vi "MDAQ_CalibrationCalcBlock.vi"(9 "threshold":dbl format="%0.2f", 10 "Spectrum":dbl[](array[numeric])) -> (1 "Mirror Fit":T1, 2 "Fit":T1, 4 "Spectrum Plot":cluster{cluster{dbl, dbl}[]}[](array[cluster]), 6 "Fitted Plots":cluster{dbl[], dbl[]}[](array[cluster]))   [LabVIEW 2021]
uses:
  <vilib>/Analysis/NI_AALPro.lvlib
  <vilib>/Analysis/NI_AAL_SigProc.lvlib
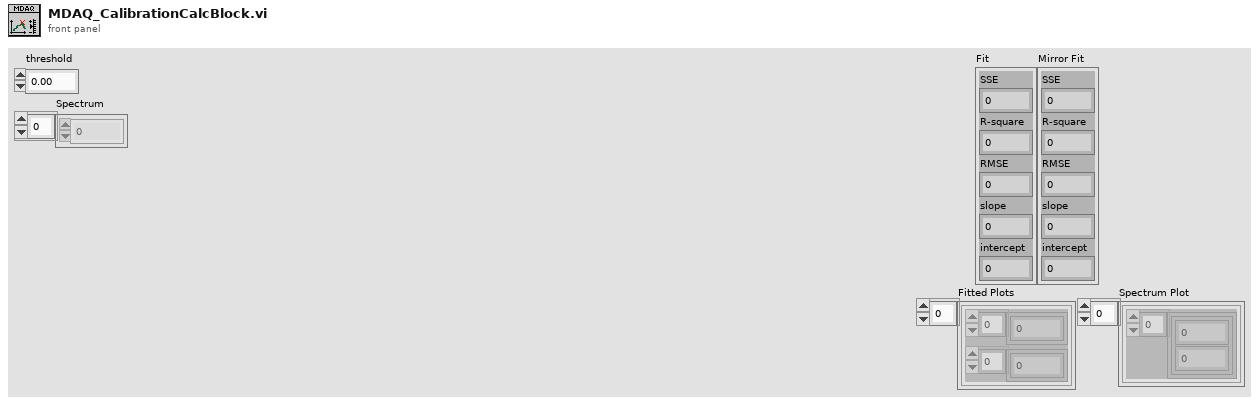
[diagram p1: front panel]
types:
  T1 = cluster{"SSE":dbl, "R-square":dbl, "RMSE":dbl, "slope":dbl, "intercept":dbl}
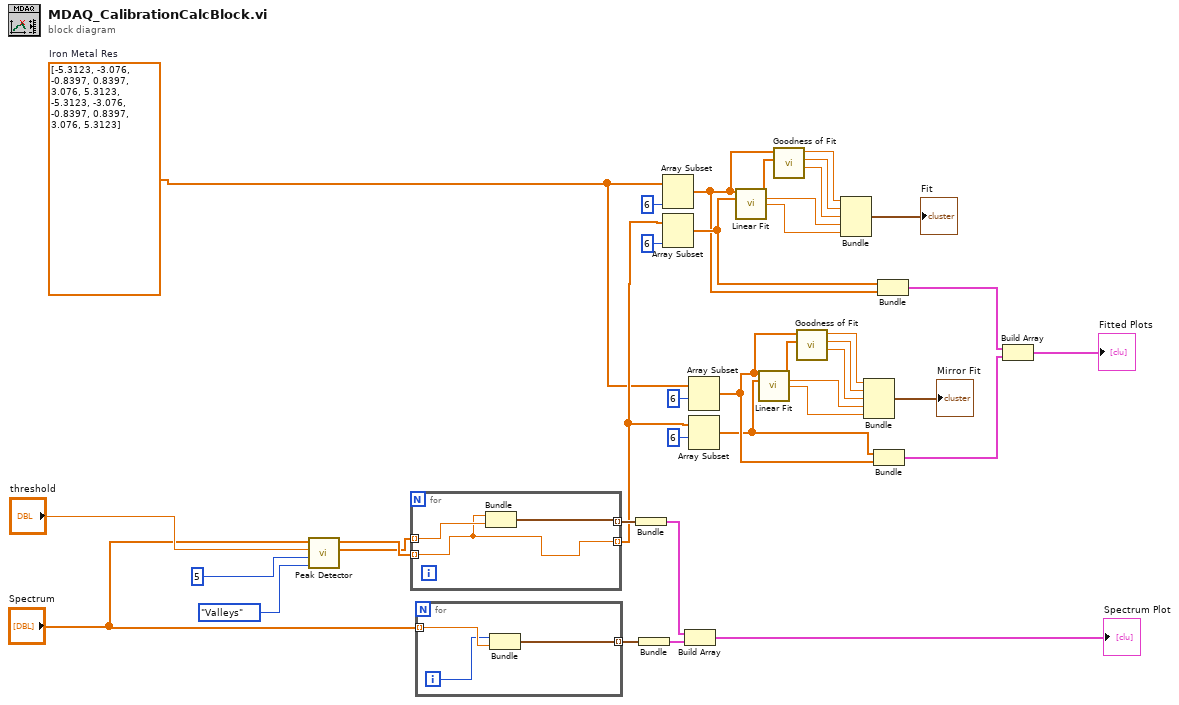
[diagram p0: block diagram]
diagram:
  w25 = dbl[] [-5.3123, -3.076, -0.8397, 0.8397, 3.076, 5.3123, -5.3123, -3.076, -0.8397, 0.8397, 3.076, 5.3123]  # Iron Metal Res
  n1 = call <vilib>:"Peak Detector.vi"("peaks/valleys"=enum32{"Peaks", "Valleys"}."Valleys", "width"=5, "threshold"="threshold", "X"="Spectrum") -> ("Amplitudes"=w35:dbl[], "Locations"=w36:dbl[])  [unwired: 3 in, 3 out]
  n2 = for {
    tunnel: w36 -> [w39] mode=indexing
    tunnel: [w39] -> w26 mode=indexing
    tunnel: w35 -> [w40] mode=indexing
    tunnel: [w41] -> w34 mode=indexing
    n3 = Bundle(w39, w40) -> (w41:cluster{dbl, dbl})  [unwired: 1 in]
  }
  n4 = for {
    tunnel: "Spectrum" -> [w44] mode=indexing
    tunnel: [w42] -> w33 mode=indexing
    i -> [w43]
    n5 = Bundle(w43, w44) -> (w42:cluster{i32, dbl})  [unwired: 1 in]
  }
  n6 = Bundle(w34) -> (w32:cluster{cluster{dbl, dbl}[]})  [unwired: 1 in]
  n7 = Bundle(w33) -> (w31:cluster{cluster{i32, dbl}[]})  [unwired: 1 in]
  n8 = Array Subset(array=w25, length=6) -> (w21:dbl[])  [unwired: 1 in]
  n9 = Array Subset(array=w26, length=6) -> (w24:dbl[])  [unwired: 1 in]
  n10 = Build Array(w32, w31) -> (→"Spectrum Plot":cluster{cluster{dbl, dbl}[]}[])
  n11 = Array Subset(array=w25, index=6) -> (w6:dbl[])  [unwired: 1 in]
  n12 = Array Subset(array=w26, index=6) -> (w5:dbl[])  [unwired: 1 in]
  n13 = call <vilib>:"Linear Fit.vi"("Y"=w21, "X"=w24) -> ("Best Linear Fit"=w20:dbl[], "slope"=w16:dbl, "intercept"=w15:dbl)  [unwired: 9 in, 2 out]
  n14 = call <vilib>:"Linear Fit.vi"("Y"=w6, "X"=w5) -> ("Best Linear Fit"=w13:dbl[], "slope"=w9:dbl, "intercept"=w8:dbl)  [unwired: 9 in, 2 out]
  n15 = call <vilib>:"Goodness of Fit.vi"("Best Fit"=w20, "Y"=w21) -> ("RMSE"=w17:dbl, "R-square"=w18:dbl, "SSE"=w19:dbl)  [unwired: 6 in, 1 out]
  n16 = call <vilib>:"Goodness of Fit.vi"("Best Fit"=w13, "Y"=w6) -> ("RMSE"=w10:dbl, "R-square"=w11:dbl, "SSE"=w12:dbl)  [unwired: 6 in, 1 out]
  n17 = Bundle("SSE"=w19, "R-square"=w18, "RMSE"=w17, "slope"=w16, "intercept"=w15) -> (→"Fit":T1)  [unwired: 1 in]
  n18 = Bundle("SSE"=w12, "R-square"=w11, "RMSE"=w10, "slope"=w9, "intercept"=w8) -> (→"Mirror Fit":T1)  [unwired: 1 in]
  n19 = Bundle(w5, w6) -> (w22:cluster{dbl[], dbl[]})  [unwired: 1 in]
  n20 = Bundle(w24, w21) -> (w23:cluster{dbl[], dbl[]})  [unwired: 1 in]
  n21 = Build Array(w23, w22) -> (→"Fitted Plots":cluster{dbl[], dbl[]}[])
